vi "Save 1 Series TDMS.vi"(6 "Sa dane?":bool, 8 "error in (no error)":errorcluster, 9 "Group Data":T3, 10 "Przebiegi in":T1, 11 "File Data":T2) -> (0 "error out":errorcluster, 2 "Przebiegi out":T1)   [LabVIEW 2014]
uses:
  Kontrolki/Przetwarzanie/Kanaly.ctl
  Kontrolki/FVGs/TDMS Group dane FVG.ctl
  Kontrolki/FVGs/TDMS File dane FVG.ctl
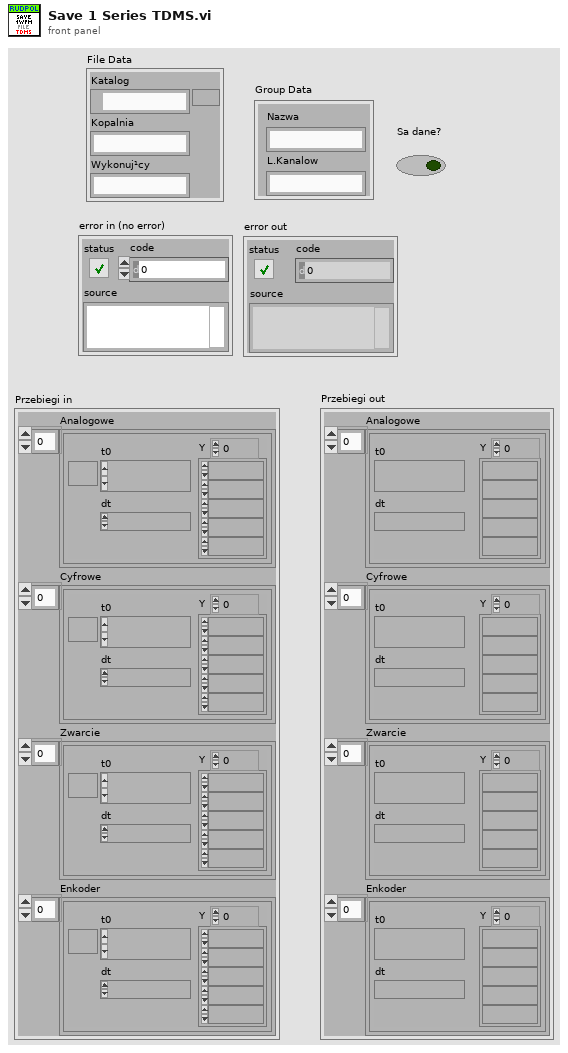
[diagram p1: front panel]
types:
  T1 = typedef "Kanaly.ctl" = cluster{"Analogowe":waveform(dbl)[], "Cyfrowe":waveform(dbl)[], "Zwarcie":waveform(dbl)[], "Enkoder":waveform(dbl)[]}
  T2 = typedef "TDMS File dane FVG.ctl" = cluster{"Katalog":path, "Kopalnia":string, "Wykonuj¹cy":string}
  T3 = typedef "TDMS Group dane FVG.ctl" = cluster{"Nazwa":string, "L.Kanalow":string}
  T4 = enum16{"open", "open or create", "create or replace", "create", "open (read-only)"}
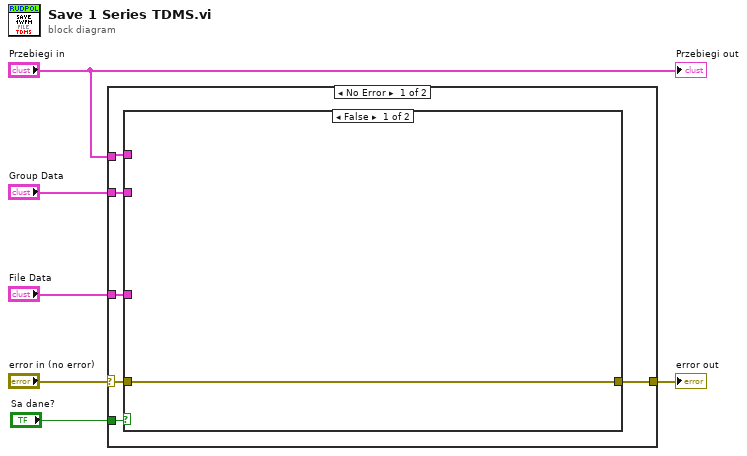
[diagram p0: block diagram]
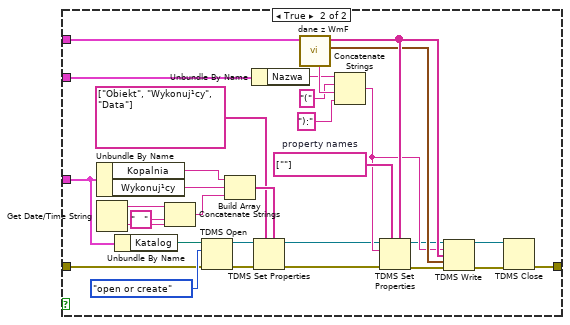
[diagram p2: hidden frame]
diagram:
  n1 = case shown="No Error" "error in (no error)" {
    selector: "error in (no error)" -> [w12 w45]
    tunnel: [w8 w45] -> w5
    tunnel: "File Data" -> [w11 _]
    tunnel: "Przebiegi in" -> [w10 _]
    tunnel: "Group Data" -> [w9 _]
    tunnel: "Sa dane?" -> [w7 _]
    frame No Error {
      n2 = case shown="False" w7 {
        tunnel: w12 -> [w13 w32]
        tunnel: w11 -> [_ w31]
        tunnel: w10 -> [_ w18]
        tunnel: w9 -> [_ w17]
        tunnel: [w13 w14] -> w8
        frame False {
        }
        frame True {
          w28 = string[] [""]  # property names
          n3 = Unbundle By Name(w31) -> ("Kopalnia"=w40:string, "Wykonuj¹cy"=w41:string)
          n4 = Get Date/Time String() -> (date string=w37:string, time string=w38:string)  [unwired: 3 in]
          n5 = Unbundle By Name(w31) -> ("Katalog"=w44:path)
          n6 = Concatenate Strings(w37, "   " ("string"), w38) -> (w42:string)
          n7 = TDMS Open(8:w32, 10:T4."open or create" ("operation (0:open)"), 11:w44) -> (0:w34:errorcluster, 3:w35:refnum<k34>)  [unwired: 4 in]
          n8 = Build Array(w40, w41, w42) -> (w43:string[])
          n9 = Unbundle By Name(w17) -> ("Nazwa"=w21:string)
          n10 = TDMS Set Properties(5:w43, 7:string[] ["Obiekt", "Wykonuj¹cy", "Data"], 8:w34, 11:w35) -> (0:w20:errorcluster, 3:w19:refnum<k34>)  [unwired: 2 in, 2 out]
          n11 = call "dane z WmF.vi"("Przebiegi in"=w18) -> ("przebiegi"=w27:waveform(dbl)[], "Nazwy"=w30:string[], "Kanaly"=w29:string)  [unwired: 6 in, 2 out]
          n12 = Concatenate Strings(w21, "(" ("string"), w29, "):" ("string")) -> (w26:string)
          n13 = TDMS Set Properties(5:w30, 7:w28, 8:w20, 10:w26, 11:w19) -> (0:w24:errorcluster, 3:w25:refnum<k34>)  [unwired: 1 in, 2 out]
          n14 = TDMS Write(0:w25, 5:w26, 7:w30, 9:w27, 11:w24) -> (4:w15:refnum<k34>, 15:w16:errorcluster)  [unwired: 1 in, 2 out]
          n15 = TDMS Close(8:w16, 11:w15) -> (0:w14:errorcluster)  [unwired: 1 out]
        }
      }
    }
    frame Error {
    }
  }
  "error out" <- w5
  "Przebiegi out" <- "Przebiegi in"
